vi "Init.vi"(8 "Error In":errorcluster, 10 "HAL.lvlib:IConfigure":refnum<class "IConfigure.lvclass">, 11 "object in":refnum<class "Scope Base.lvclass">) -> (0 "Error Out":errorcluster, 3 "object out":refnum<class "Scope Base.lvclass">)   [LabVIEW 2023, in "Scope Base.lvlib" / "Scope Base.lvclass"]
uses:
  Scope Base.lvclass
  Scope Base.lvclass/Scope Base.ctl
  Interfaces/IConfigure Scope/IConfigure Scope.lvclass
  Interfaces/IConfigure/IConfigure.lvclass
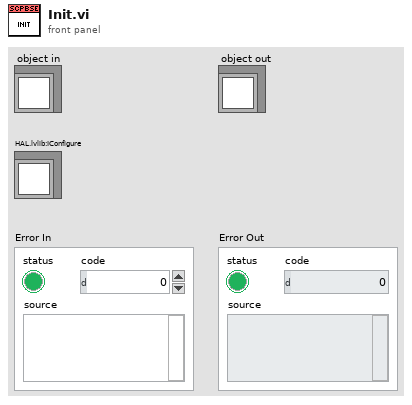
[diagram p1: front panel]
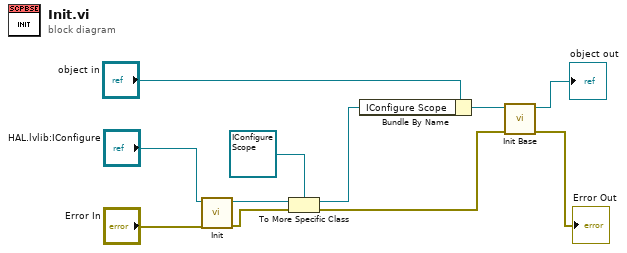
[diagram p0: block diagram]
diagram:
  n1 = call-dynamic "Init.vi"("error in (no error)"="Error In", "IConfigure in"="HAL.lvlib:IConfigure") -> ("error out"=w5:errorcluster, "IConfigure out"=w10:refnum<class "IConfigure.lvclass">)  [unwired: 8 in]
  n2 = To More Specific Class(target class=refnum<class "IConfigure Scope.lvclass"> refnum ("IConfigure Scope.lvclass"), reference=w10, error in=w5) -> (specific class reference=w7:refnum<class "IConfigure Scope.lvclass">, error out=w4:errorcluster)
  n3 = Bundle By Name(cluster="object in", "IConfigure Scope"=w7) -> (w2:refnum<class "Scope Base.lvclass">)
  n4 = call-dynamic "Init Base.vi"("Error In"=w4, "object in"=w2) -> ("Error Out"=→"Error Out":errorcluster, "object out"=→"object out":refnum<class "Scope Base.lvclass">)  [unwired: 8 in]
